vi "MGCC_DataLog_sub.vi"() -> ()   [LabVIEW 2016]
uses:
  Finite State Machine/Sub-VIs/MGCC_FntStaMach_gobal.vi
panel:
  in  "Start 4":bool=TRUE
  out "error out 2":errorcluster
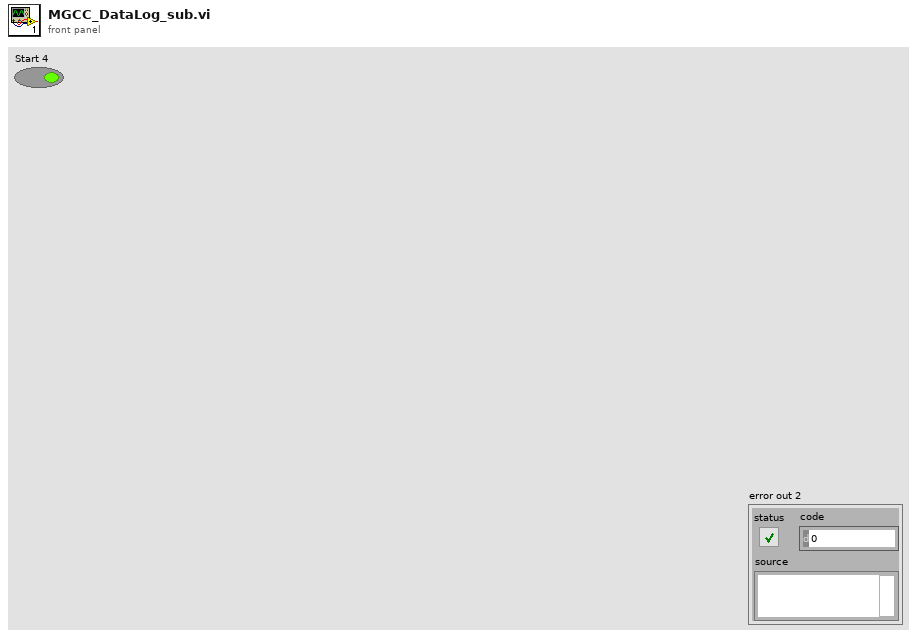
[diagram p1: front panel]
types:
  T1 = enum16{"open", "open or create", "create or replace", "create", "open (read-only)"}
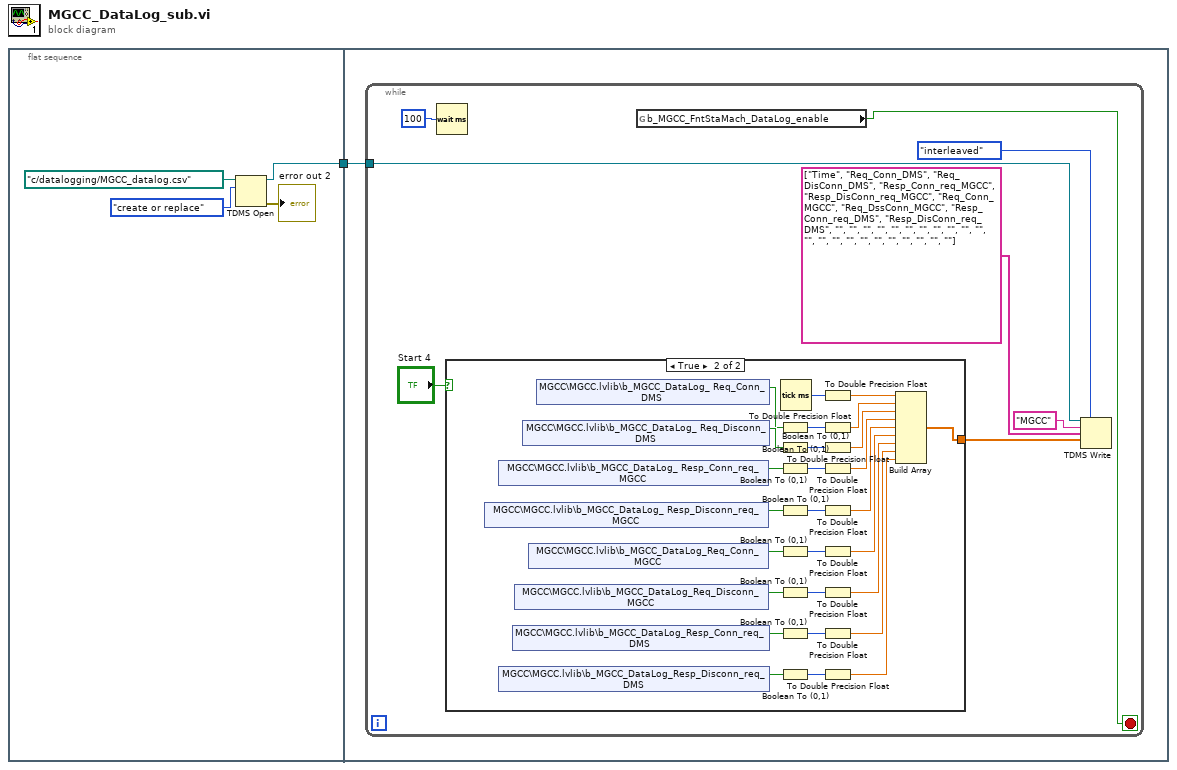
[diagram p0: block diagram]
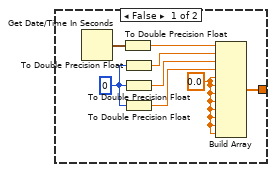
[diagram p2: hidden frame]
diagram:
  n1 = flat-sequence {
    tunnel: [w4] -> w1
    tunnel: w1 -> [w6]
    frame #0 {
      n2 = TDMS Open(10:T1."create or replace" ("operation (0:open)"), 11:path "c:/datalogging/MGCC_datalog.csv" ("file path (dialog if empty)")) -> (0:→"error out 2":errorcluster, 3:w4:refnum<k34>)  [unwired: 5 in]
    }
    frame #1 {
      n3 = while {
        tunnel: w6 -> [w9]
        stop <- w7 stop-if-true
        n4 = Wait (ms)(milliseconds to wait=u32 100) -> ()  [unwired: 1 out]
        n5 = case shown="True" "Start 4" {
          tunnel: [w15 w48] -> w11
          frame False {
            w17 = 0.0
            w21 = 0
            n6 = Get Date/Time In Seconds() -> (seconds since 1Jan1904=w22:timestamp)
            n7 = To Double Precision Float(number=w22) -> (double precision float=w20:dbl)
            n8 = To Double Precision Float(number=w21) -> (double precision float=w16:dbl)
            n9 = To Double Precision Float(number=w21) -> (double precision float=w18:dbl)
            n10 = To Double Precision Float(number=w21) -> (double precision float=w19:dbl)
            n11 = Build Array(w20, w16, w18, w19, w17, w17, w17, w17, w17, w17, w17, w17) -> (w15:dbl[])
          }
          frame True {
            n12 = shared-variable "MGCC\\MGCC.lvlib\\b_MGCC_DataLog_ Resp_Disconn_req_MGCC"() -> (w36:bool)  [unwired: 1 in, 1 out]
            n13 = shared-variable "MGCC\\MGCC.lvlib\\b_MGCC_DataLog_ Resp_Conn_req_MGCC"() -> (w35:bool)  [unwired: 1 in, 1 out]
            n14 = shared-variable "MGCC\\MGCC.lvlib\\b_MGCC_DataLog_Resp_Disconn_req_DMS"() -> (w39:bool)  [unwired: 1 in, 1 out]
            n15 = shared-variable "MGCC\\MGCC.lvlib\\b_MGCC_DataLog_Resp_Conn_req_DMS"() -> (w38:bool)  [unwired: 1 in, 1 out]
            n16 = shared-variable "MGCC\\MGCC.lvlib\\b_MGCC_DataLog_Req_Disconn_MGCC"() -> (w37:bool)  [unwired: 1 in, 1 out]
            n17 = shared-variable "MGCC\\MGCC.lvlib\\b_MGCC_DataLog_ Req_Disconn_DMS"() -> (w34:bool)  [unwired: 1 in, 1 out]
            n18 = shared-variable "MGCC\\MGCC.lvlib\\b_MGCC_DataLog_Req_Conn_MGCC"() -> (w33:bool)  [unwired: 1 in, 1 out]
            n19 = shared-variable "MGCC\\MGCC.lvlib\\b_MGCC_DataLog_ Req_Conn_DMS"() -> (w32:bool)  [unwired: 1 in, 1 out]
            n20 = Boolean To (0,1)(Boolean=w32) -> (0, 1=w47:i16)
            n21 = Boolean To (0,1)(Boolean=w34) -> (0, 1=w46:i16)
            n22 = Boolean To (0,1)(Boolean=w35) -> (0, 1=w45:i16)
            n23 = Boolean To (0,1)(Boolean=w36) -> (0, 1=w44:i16)
            n24 = Boolean To (0,1)(Boolean=w33) -> (0, 1=w43:i16)
            n25 = Boolean To (0,1)(Boolean=w37) -> (0, 1=w42:i16)
            n26 = Boolean To (0,1)(Boolean=w38) -> (0, 1=w41:i16)
            n27 = Boolean To (0,1)(Boolean=w39) -> (0, 1=w40:i16)
            n28 = Tick Count (ms)() -> (millisecond timer value=w49:u32)
            n29 = To Double Precision Float(number=w49) -> (double precision float=w31:dbl)
            n30 = To Double Precision Float(number=w47) -> (double precision float=w30:dbl)
            n31 = To Double Precision Float(number=w46) -> (double precision float=w29:dbl)
            n32 = To Double Precision Float(number=w45) -> (double precision float=w28:dbl)
            n33 = To Double Precision Float(number=w44) -> (double precision float=w27:dbl)
            n34 = To Double Precision Float(number=w43) -> (double precision float=w26:dbl)
            n35 = To Double Precision Float(number=w42) -> (double precision float=w25:dbl)
            n36 = To Double Precision Float(number=w41) -> (double precision float=w24:dbl)
            n37 = To Double Precision Float(number=w40) -> (double precision float=w23:dbl)
            n38 = Build Array(w31, w30, w29, w28, w27, w26, w25, w24, w23) -> (w48:dbl[])
          }
        }
        n39 = global read "MGCC_FntStaMach_gobal.vi" "b_MGCC_FntStaMach_DataLog_enable"() -> (w7:bool)
        n40 = TDMS Write(0:w9, 1:enum16{"decimated", "interleaved"}."interleaved" ("data layout (0:decimated)"), 5:"MGCC" ("group name in (Untitled)"), 7:string[] ["Time", "Req_Conn_DMS", "Req_DisConn_DMS", "Resp_Conn_req_MGCC", "Resp_DisConn_req_MGCC", "Req_Conn_MGCC", "Req_DssConn_MGCC", "Resp_Conn_req_DMS", "Resp_DisConn_req_DMS", "", "", "", "", "", "", "", "", "", "", "", "", "", "", "", "", "", "", "", "", "", ""] ("channel name(s) in (Untitled)"), 9:w11) -> ()  [unwired: 1 in, 4 out]
      }
    }
  }
